vi "Main.vi"() -> ()   [LabVIEW 2012]
uses:
  Consumer Message.ctl
  <vilib>/Utility/error.llb/Error Cluster From Error Code.vi
  <vilib>/ErrorRing/Error Ring.xnode
panel:
  in  "Producer Error":bool
  in  "Consumer Error":bool
  out "Consumer Shutdown?":bool
  out "State to Execute":string
  out "High Priority?":bool
  out "Backlog":u8(slide) scale=0.0..100.0
  out "Processed Value":i32
  in  "High Priority Message":bool
  in  "Normal Priority Message":bool
  in  "Stop":bool
  # "Number of enqueued\nmessages waiting to\nbe processed"
  # "Current data being\nprocessed in consumer loop"
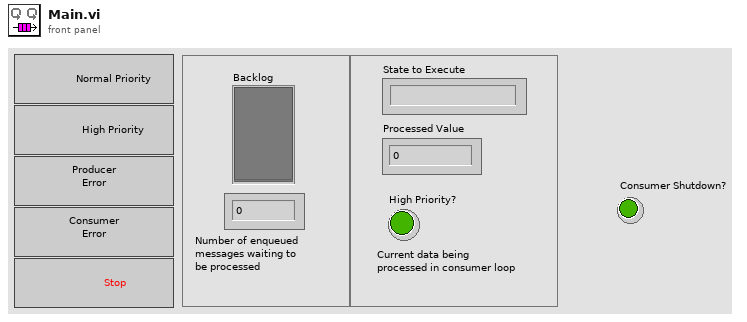
[diagram p1: front panel]
types:
  T1 = typedef "Consumer Message.ctl" = cluster{"Consumer State":string, "Boolean Data":bool, "Numeric Data":i32, "Error":errorcluster}
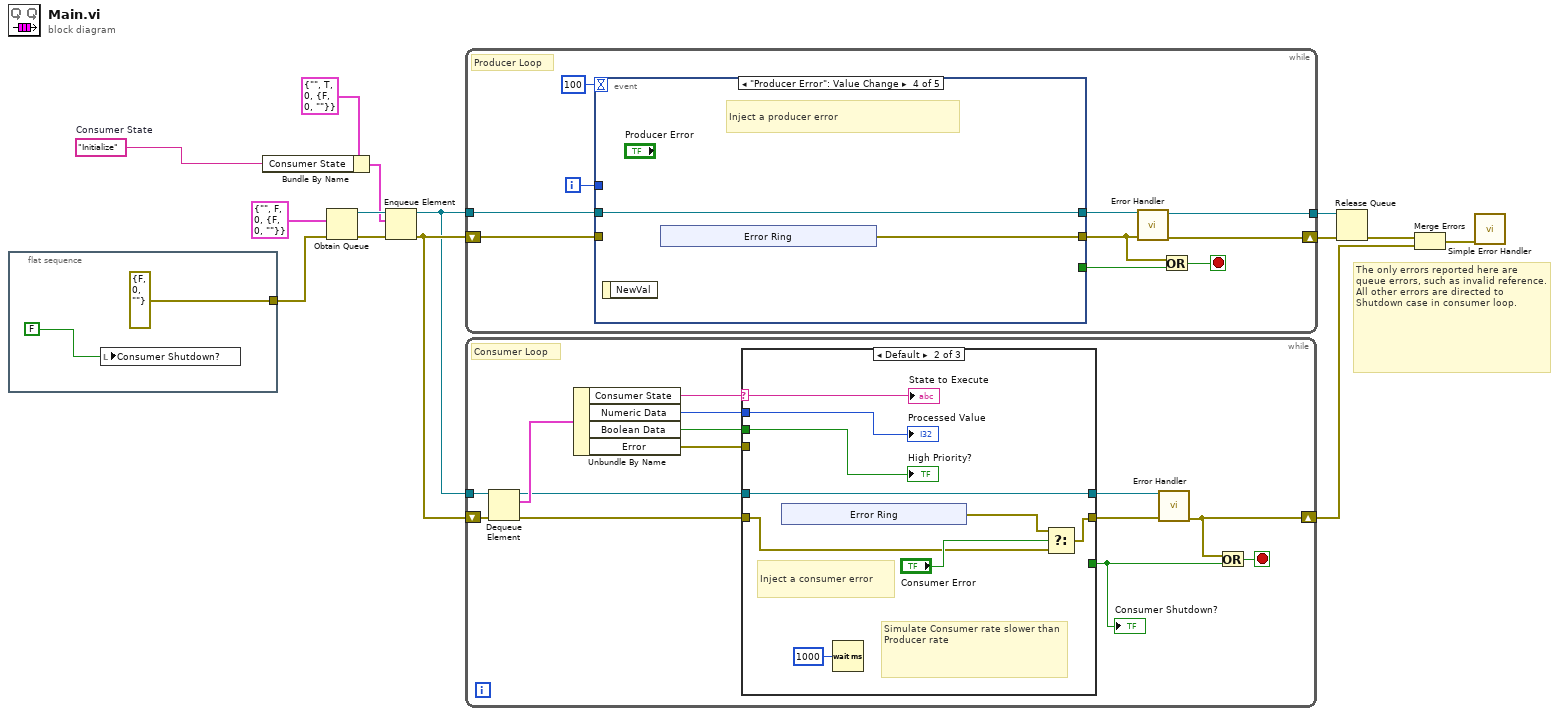
[diagram p0: block diagram]
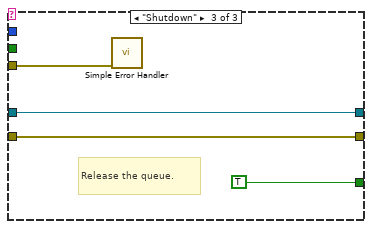
[diagram p3: hidden frame]
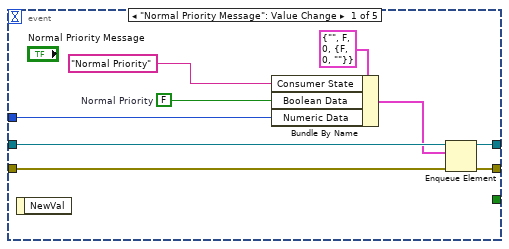
[diagram p4: hidden frame]
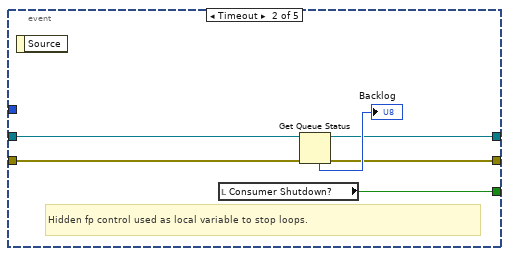
[diagram p5: hidden frame]
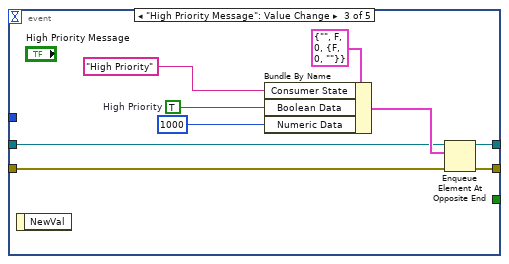
[diagram p6: hidden frame]
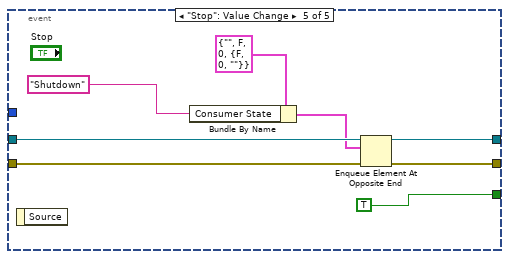
[diagram p7: hidden frame]
diagram:
  w6 = "Initialize"  # Consumer State
  # "The only errors reported here are queue errors, such as invalid reference.  All other errors are directed to Shutdown case in consumer loop."
  n1 = flat-sequence {
    tunnel: [errorcluster {"status"=FALSE, "code"=0, "source"=""} ("error in (no error)")] -> w9
    frame #0 {
      n2 = local write "Consumer Shutdown?"(FALSE ("Stop Loops (local)")) -> ()
    }
  }
  n3 = Bundle By Name(cluster=T1 {"Consumer State"="", "Boolean Data"=TRUE, "Numeric Data"=0, "Error"={"status"=FALSE, "code"=0, "source"=""}} ("Consumer Message"), "Consumer State"=w6) -> (w7:T1)
  n4 = Obtain Queue(element data type=T1 {"Consumer State"="", "Boolean Data"=FALSE, "Numeric Data"=0, "Error"={"status"=FALSE, "code"=0, "source"=""}}, error in (no error)=w9) -> (queue out=w11:refnum<queue>, error out=w14:errorcluster)  [unwired: 3 in, 1 out]
  n5 = Enqueue Element(queue=w11, element=w7, error in (no error)=w14) -> (queue out=w10:refnum<queue>, error out=w12:errorcluster)  [unwired: 1 in, 1 out]
  n6 = while {
    tunnel: w10 -> [w26]
    shift-right: [w18] -> w4
    shift-left: w12 -> [w25]
    tunnel: [w17] -> w3
    i -> [w24]
    stop <- w20 stop-if-true
    # "Producer Loop"
    n7 = event shown="[3] \"Producer Error\": Value Change" {
      selector: _ -> [_ _ _ _ _]
      dyn-events: _ -> [_ _ _ _ _]
      timeout: 100 -> [_ _ _ _ _]
      tunnel: w26 -> [w35 w39 w42 w51 w64]
      tunnel: w25 -> [w33 w38 w49 _ w62]
      tunnel: [w34 w37 w50 w52 w61] -> w19
      tunnel: [_ w41 _ _ TRUE] -> w21
      tunnel: w24 -> [w32 _ _ _ _]
      tunnel: [w28 w36 w45 w51 w60] -> w23
      event "Normal Priority Message": Value Change {
        w29 = FALSE  # Normal Priority
        n8 = event-data() -> ()  [unwired: 1 in, 1 out]
        n9 = Bundle By Name(cluster=T1 {"Consumer State"="", "Boolean Data"=FALSE, "Numeric Data"=0, "Error"={"status"=FALSE, "code"=0, "source"=""}}, "Consumer State"="Normal Priority" ("String Data"), "Boolean Data"=w29, "Numeric Data"=w32) -> (w31:T1)
        n10 = Enqueue Element(queue=w35, element=w31, error in (no error)=w33) -> (queue out=w28:refnum<queue>, error out=w34:errorcluster)  [unwired: 1 in, 1 out]
      }
      event Timeout {
        # "Hidden fp control used as local variable to stop loops."
        n11 = event-data() -> ()  [unwired: 1 in, 1 out]
        n12 = local read "Consumer Shutdown?"() -> (w41:bool)
        n13 = Get Queue Status(queue=w39, error in (no error)=w38) -> (queue out=w36:refnum<queue>, error out=w37:errorcluster, # elements in queue=→"Backlog":i32)  [unwired: 1 in, 5 out]
      }
      event "High Priority Message": Value Change {
        w44 = TRUE  # High Priority
        n14 = event-data() -> ()  [unwired: 1 in, 1 out]
        n15 = Bundle By Name(cluster=T1 {"Consumer State"="", "Boolean Data"=FALSE, "Numeric Data"=0, "Error"={"status"=FALSE, "code"=0, "source"=""}}, "Consumer State"="High Priority" ("String Data"), "Boolean Data"=w44, "Numeric Data"=1000) -> (w47:T1)
        n16 = Enqueue Element At Opposite End(queue=w42, element=w47, error in (no error)=w49) -> (queue out=w45:refnum<queue>, error out=w50:errorcluster)  [unwired: 1 in, 1 out]
      }
      event "Producer Error": Value Change {
        # "Inject a producer error"
        n17 = event-data() -> ()  [unwired: 1 in, 1 out]
        n18 = xnode "Error Ring"() -> ("error out"=w52:errorcluster)
      }
      event "Stop": Value Change {
        n19 = event-data() -> ()  [unwired: 1 in, 1 out]
        n20 = Bundle By Name(cluster=T1 {"Consumer State"="", "Boolean Data"=FALSE, "Numeric Data"=0, "Error"={"status"=FALSE, "code"=0, "source"=""}}, "Consumer State"="Shutdown") -> (w57:T1)
        n21 = Enqueue Element At Opposite End(queue=w64, element=w57, error in (no error)=w62) -> (queue out=w60:refnum<queue>, error out=w61:errorcluster)  [unwired: 1 in, 1 out]
      }
    }
    n22 = call "Error Handler.vi"("error in"=w19, "queue in"=w23) -> ("error out"=w18:errorcluster, "queue out"=w17:refnum<queue>)  [unwired: 8 in]
    n23 = Or(x=w19, y=w21) -> (x .or. y?=w20:bool)
  }
  n24 = while {
    tunnel: w10 -> [w78]
    shift-right: [w67] -> w1
    shift-left: w12 -> [w77]
    stop <- w68 stop-if-true
    # "Consumer Loop"
    n25 = Dequeue Element(queue=w78, error in (no error)=w77) -> (queue out=w66:refnum<queue>, element=w76:T1, error out=w65:errorcluster)  [unwired: 1 in, 1 out]
    n26 = Unbundle By Name(w76) -> ("Consumer State"=w75:string, "Numeric Data"=w74:i32, "Boolean Data"=w73:bool, "Error"=w70:errorcluster)
    n27 = case shown="Default" w75 {
      selector: w75 -> [_ w86 _]
      tunnel: [_ _ TRUE] -> w69
      tunnel: w65 -> [w79 w82 w95]
      tunnel: [w79 w83 w95] -> w72
      tunnel: w74 -> [_ w89 _]
      tunnel: w73 -> [_ w88 _]
      tunnel: w66 -> [w80 w87 w96]
      tunnel: [w80 w87 w96] -> w71
      tunnel: w70 -> [_ _ w97]
      frame "Initialize" {
      }
      frame Default {
        # "Inject a consumer error"
        # "Simulate Consumer rate slower than Producer rate"
        n28 = xnode "Error Ring"() -> ("error out"=w81:errorcluster)
        n29 = Wait (ms)(milliseconds to wait=u32 1000) -> ()  [unwired: 1 out]
        n30 = Select(t=w81, s="Consumer Error", f=w82) -> (s? t:f=w83:errorcluster)
        "Processed Value" <- w89
        "High Priority?" <- w88
        "State to Execute" <- w86
      }
      frame "Shutdown" {
        # "Release the queue."
        n31 = call <vilib>:"Simple Error Handler.vi"("error in (no error)"=w97) -> ()  [unwired: 4 in, 5 out]
      }
    }
    "Consumer Shutdown?" <- w69
    n32 = call "Error Handler.vi"("error in"=w72, "queue in"=w71) -> ("error out"=w67:errorcluster)  [unwired: 8 in, 1 out]
    n33 = Or(x=w67, y=w69) -> (x .or. y?=w68:bool)
  }
  n34 = Release Queue(queue=w3, error in (no error)=w4) -> (error out=w2:errorcluster)  [unwired: 1 in, 2 out]
  n35 = Merge Errors(w2, w1) -> (w5:errorcluster)
  n36 = call <vilib>:"Simple Error Handler.vi"("error in (no error)"=w5) -> ()  [unwired: 4 in, 5 out]
